vi "Get Tags of All Child Items.vi"(8 "error in":errorcluster, 10 "Parent Tag":string, 11 "Tree Ref in":refnum<vi>) -> (0 "error out":errorcluster, 1 "Tags of All Child Items":string[](array[string]), 2 "Parent Tag Out":string, 3 "Tree Ref Out":refnum<vi>, 4 "Children Found?":bool)   [LabVIEW 2013, in "LVTM.lvlib"]
uses:
  LVTM.lvlib
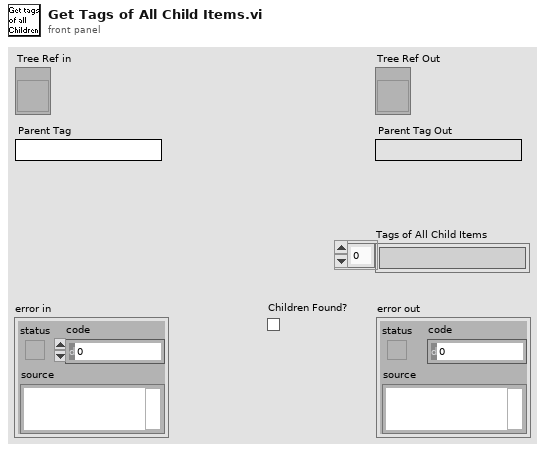
[diagram p1: front panel]
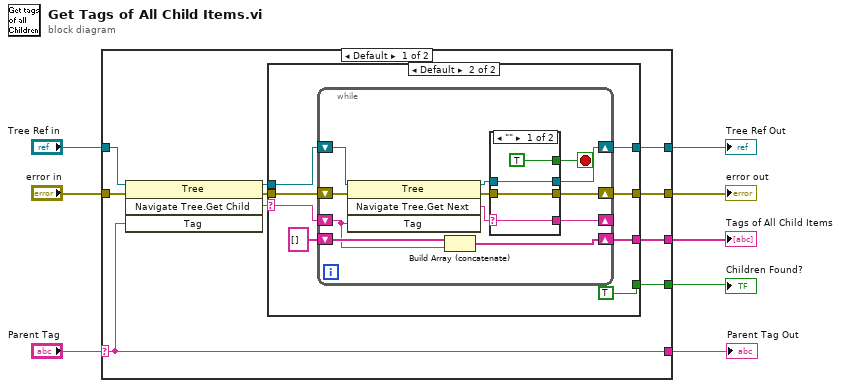
[diagram p0: block diagram]
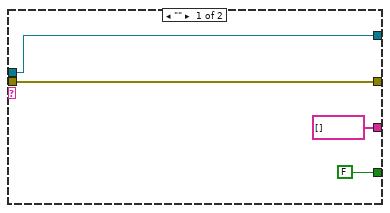
[diagram p2: hidden frame]
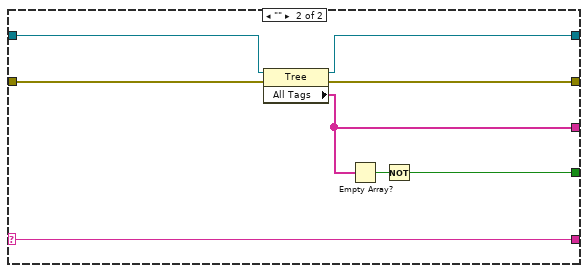
[diagram p4: hidden frame]
diagram:
  n1 = case shown="Default" "Parent Tag" {
    selector: "Parent Tag" -> [w9 w53]
    tunnel: [w18 w52] -> w8
    tunnel: [w17 w55] -> w7
    tunnel: "error in" -> [w16 w57]
    tunnel: "Tree Ref in" -> [w15 w56]
    tunnel: [w12 w54] -> w4
    tunnel: [w10 w50] -> w3
    tunnel: [w9 w53] -> w1
    frame Default {
      n2 = invoke class="Tree" method="Navigate Tree.Get Child"(reference=w15, error in=w16, "Tag"=w9) -> (reference out=w14:refnum<vi>, error out=w13:errorcluster, "Navigate Tree:Get Child"=w11:string)  [unwired: 1 in, 1 out]
      n3 = case shown="Default" w11 {
        selector: w11 -> [_ w24]
        tunnel: [string[] [] w30] -> w18
        tunnel: [w21 w29] -> w17
        tunnel: w14 -> [w22 w28]
        tunnel: w13 -> [w21 w27]
        tunnel: [w22 w26] -> w12
        tunnel: [FALSE ("Children Found?") TRUE ("Children Found?")] -> w10
        frame "" {
        }
        frame Default {
          n4 = while {
            shift-right: [w37] -> w29
            shift-left: w27 -> [w42]
            shift-right: [w38] -> w26
            shift-left: w28 -> [w41]
            shift-right: [w36] -> _
            shift-left: w24 -> [w31]
            shift-right: [w32] -> w30
            shift-left: string[] [] -> [w33]
            stop <- w34 stop-if-true
            n5 = invoke class="Tree" method="Navigate Tree.Get Next"(reference=w41, error in=w42, "Tag"=w31) -> (reference out=w39:refnum<vi>, error out=w40:errorcluster, "Navigate Tree:Get Next Item"=w35:string)  [unwired: 1 in, 1 out]
            n6 = Build Array (concatenate)(w33, w31) -> (w32:string[])
            n7 = case shown="\"\"" w35 {
              selector: w35 -> [w43 w47]
              tunnel: w40 -> [w46 w48]
              tunnel: w39 -> [w45 w49]
              tunnel: [w45 w49] -> w38
              tunnel: [w46 w48] -> w37
              tunnel: [w43 w47] -> w36
              tunnel: [TRUE _] -> w34
              frame "" {
              }
              frame Default {
              }
            }
          }
        }
      }
    }
    frame "" {
      n8 = property class="Tree"(reference=w56, error in=w57) -> (reference out=w54:refnum<vi>, error out=w55:errorcluster, "All Tags"=w52:string[])
      n9 = Empty Array?(array=w52) -> (empty?=w51:bool)
      n10 = Not(x=w51) -> (.not. x?=w50:bool)
    }
  }
  "Tags of All Child Items" <- w8
  "error out" <- w7
  "Parent Tag Out" <- w1
  "Tree Ref Out" <- w4
  "Children Found?" <- w3
